vi "SeverGlobal.vi"() -> ()   [LabVIEW 2015]
panel:
  out "config":T1
  in  "通道数":enum16{"64X4", "128X4"}(ring)
  out "OUT8":bool
  out "OUT7":bool
  out "OUT6":bool
  out "OUT5":bool
  out "OUT4":bool
  out "OUT3":bool
  out "OUT2":bool
  out "OUT1":bool
  out "CLK8":i32
  out "CLK7":i32
  out "CLK6":i32
  out "CLK5":i32
  out "CLK4":i32
  out "CLK3":i32
  out "CLK2":i32
  out "CLK1":i32
  in  "Broadcast":cluster{"消息类型":string, "广播？":bool}
  out "stop":bool
  out "RF4":i32
  out "RF3":i32
  out "RF2":i32
  out "RF1":i32
  in  "Timequeue":T2
  out "memebers":i32
  out "COM4":bool
  out "COM3":bool
  out "COM2":bool
  out "COM1":bool
  in  "TCP_CLK":refnum<k5>
  in  "TCP_Switch8X4":refnum<k5>
  in  "TCP_RF_B":refnum<k5>
  in  "TCP_RF_A":refnum<k5>
  in  "CLK_Waits":T3(array[cluster])
  in  "CLK_Nows":T3(array[cluster])
  in  "RF_Waits":T4(array[cluster])
  in  "RF_Nows":T4(array[cluster])
  in  "Clients":T5(array[cluster])
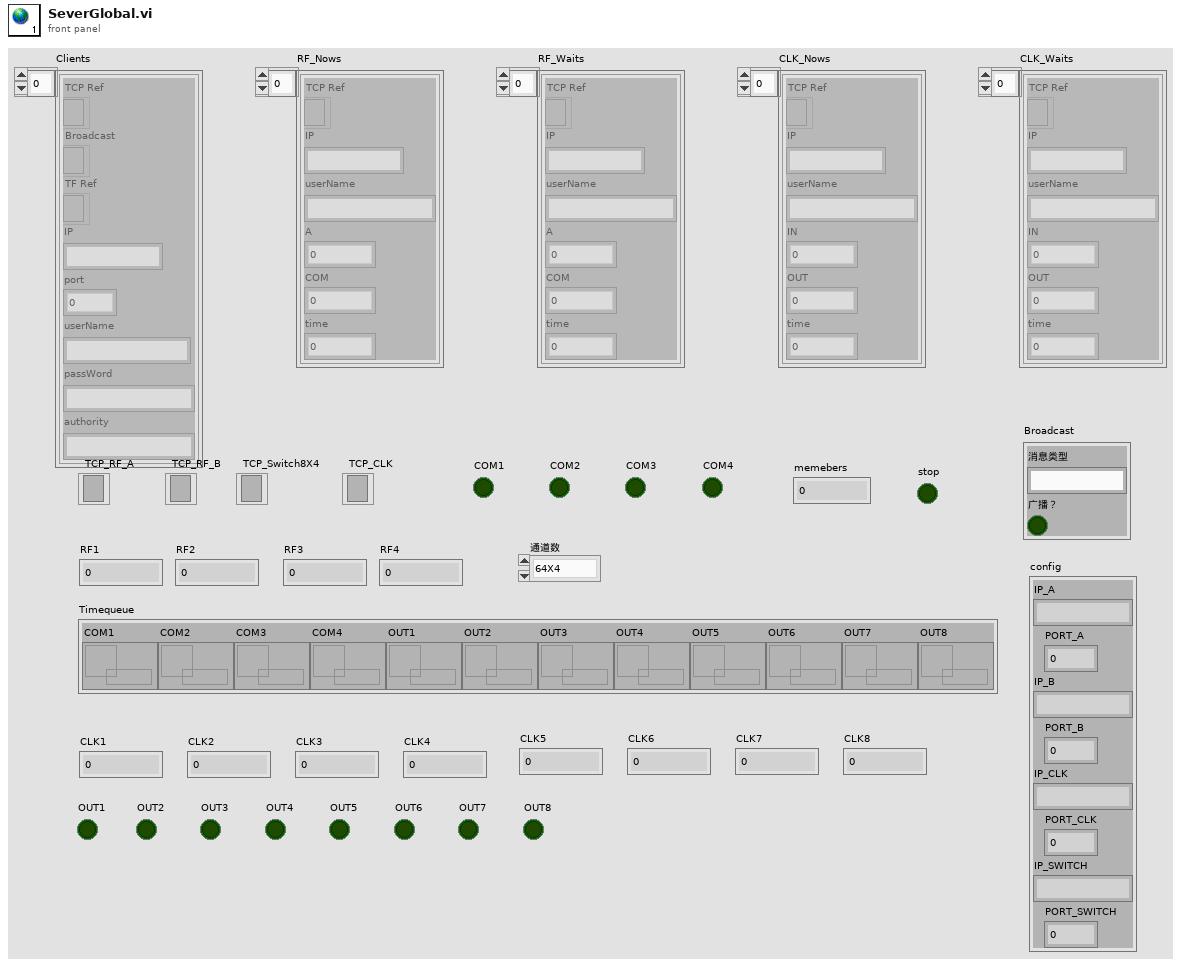
[diagram p1: front panel]
types:
  T1 = cluster{"IP_A":string, "PORT_A":i32, "IP_B":string, "PORT_B":i32, "IP_CLK":string, "PORT_CLK":i32, "IP_SWITCH":string, "PORT_SWITCH":i32}
  T2 = typedef "队列.ctl" = cluster{"COM1":refnum<queue>, "COM2":refnum<queue>, "COM3":refnum<queue>, "COM4":refnum<queue>, "OUT1":refnum<queue>, "OUT2":refnum<queue>, "OUT3":refnum<queue>, "OUT4":refnum<queue>, "OUT5":refnum<queue>, "OUT6":refnum<queue>, "OUT7":refnum<queue>, "OUT8":refnum<queue>}
  T3 = cluster{"TCP Ref":refnum<k5>, "IP":string, "userName":string, "IN":u16, "OUT":u16, "time":u32}[]
  T4 = cluster{"TCP Ref":refnum<k5>, "IP":string, "userName":string, "A":u16, "COM":u16, "time":u32}[]
  T5 = cluster{"TCP Ref":refnum<k5>, "Broadcast":refnum<k5>, "TF Ref":refnum<k5>, "IP":string, "port":u16, "userName":string, "passWord":string, "authority":string}[]
diagram:
